vi "Configure.vi"(8 "error in":errorcluster, 10 "configuration":T1, 11 "session in":T2) -> (0 "error out":errorcluster)   [LabVIEW 2021, in "dcvmDPI_AD7606B_serverImpl.lvlib"]
uses:
  dcvmDPI_AD7606B_serverImpl.lvlib
  controls/session.ctl
  controls/configuration.ctl
  <vilib>/Utility/error.llb/Error Cluster From Error Code.vi
  <vilib>/rvi/errors/niLvFpgaAdjustHostInterfaceError.vi
  <vilib>/rvi/interface/nirviReadWriteControl/nirviReadWriteControl.xnode
  NiFpgaLv.dll
  <vilib>/rvi/interface/Simulation/niFpgaSimulationCallBeginRW.vi
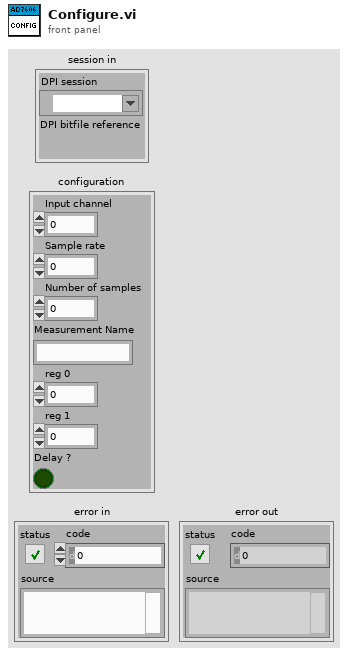
[diagram p1: front panel]
types:
  T1 = typedef "dcvmDPI_AD7606B_serverImpl.lvlib/configuration.ctl" = cluster{"Input channel":i32, "Sample rate":dbl, "Number of samples":u32, "Measurement Name":string, "reg 0":i32, "reg 1":i32, "Delay ?":bool}
  T2 = typedef "dcvmDPI_AD7606B_serverImpl.lvlib/session.ctl" = cluster{"DPI session":refnum<k15>, "DPI bitfile reference":refnum<k20>}
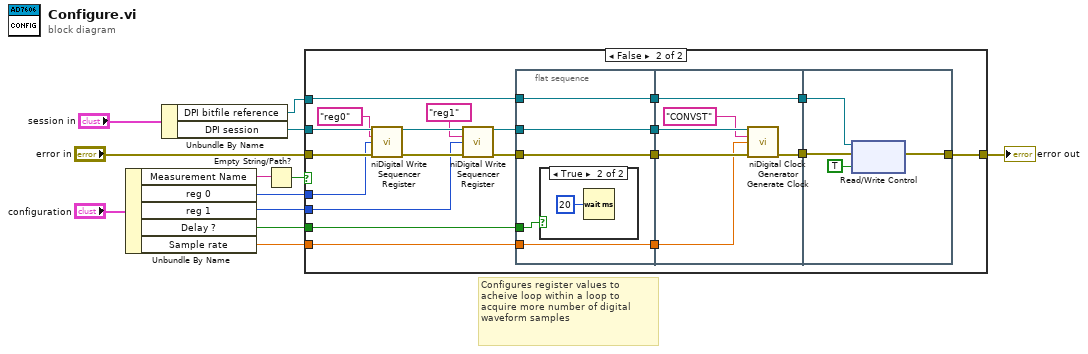
[diagram p0: block diagram]
diagram:
  # "Configures register values to acheive loop within a loop to acquire more number of digital waveform samples"
  n1 = Unbundle By Name("configuration") -> ("Measurement Name"=w2:string, "reg 0"=w5:i32, "reg 1"=w7:i32, "Delay ?"=w4:bool, "Sample rate"=w6:dbl)
  n2 = Unbundle By Name("session in") -> ("DPI bitfile reference"=w3:refnum<k20>, "DPI session"=w11:refnum<k15>)
  n3 = Empty String/Path?(string/path=w2) -> (empty?=w1:bool)
  n4 = case shown="False" w1 {
    tunnel: "error in" -> [w13 w30]
    tunnel: w11 -> [_ w33]
    tunnel: w5 -> [_ w27]
    tunnel: [w13 w22] -> w9
    tunnel: w7 -> [_ w26]
    tunnel: w6 -> [_ w20]
    tunnel: w4 -> [_ w21]
    tunnel: w3 -> [_ w18]
    frame True {
    }
    frame False {
      n5 = call <instrlib>:"niDigital Write Sequencer Register.vi"("instrument handle"=w33, "sequencer register"="reg0", "value"=w27, "error in"=w30) -> ("instrument handle out"=w32:refnum<k15>, "error out"=w31:errorcluster)  [unwired: 10 in]
      n6 = call <instrlib>:"niDigital Write Sequencer Register.vi"("instrument handle"=w32, "sequencer register"="reg1", "value"=w26, "error in"=w31) -> ("instrument handle out"=w17:refnum<k15>, "error out"=w25:errorcluster)  [unwired: 10 in]
      n7 = flat-sequence {
        tunnel: w25 -> [w37]
        tunnel: [w37] -> w23
        tunnel: w21 -> [w38]
        tunnel: w20 -> [w36]
        tunnel: [w36] -> w19
        tunnel: w18 -> [w34]
        tunnel: w17 -> [w35]
        tunnel: [w35] -> w16
        tunnel: [w34] -> w15
        tunnel: [w43] -> w24
        tunnel: w23 -> [w44]
        tunnel: w19 -> [w41]
        tunnel: w16 -> [w45]
        tunnel: w15 -> [w40]
        tunnel: [w40] -> w14
        tunnel: [w47] -> w22
        tunnel: w24 -> [w49]
        tunnel: w14 -> [w48]
        frame #0 {
          n8 = case shown="True" w38 {
            frame False {
            }
            frame True {
              n9 = Wait (ms)(milliseconds to wait=u32 20) -> ()  [unwired: 1 out]
            }
          }
        }
        frame #1 {
          n10 = call <instrlib>:"niDigital Clock Generator Generate Clock.vi"("instrument handle"=w45, "channel list"="CONVST", "frequency (Hz)"=w41, "error in"=w44) -> ("error out"=w43:errorcluster)  [unwired: 10 in, 1 out]
        }
        frame #2 {
          n11 = xnode "Read/Write Control"("FPGA VI Reference In"=w48, "error in"=w49, "active"=TRUE) -> ("error out"=w47:errorcluster)  [unwired: 1 out]
        }
      }
    }
  }
  "error out" <- w9
